vi "CRYImp wiz load settings.vi"() -> (0 "error out":errorcluster, 1 "Canceled":bool, 2 "x-y settings array out":T1 {"yp db ref" format="%.2f"; "ym db ref" format="%.2f"; "x db ref" format="%.2f"}, 3 "Main info cluster out":T2)   [LabVIEW 2013]
uses:
  Control/CRYImp wiz main info.ctl
  Control/CRYx-y settings array.ctl
  CRYMainGlobal.vi
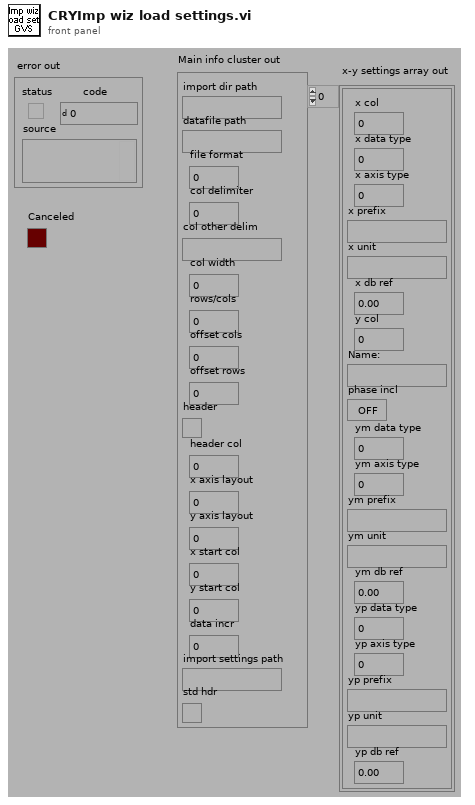
[diagram p1: front panel]
types:
  T1 = typedef "CRYx-y settings array.ctl" = cluster{"x col":i32, "x data type":u16, "x axis type":u16, "x prefix":string, "x unit":string, "x db ref":dbl, "y col":i32, "Name:":string, "phase incl":bool, "ym data type":u16, "ym axis type":u16, "ym prefix":string, "ym unit":string, "ym db ref":dbl, "yp data type":u16, "yp axis type":u16, "yp prefix":string, "yp unit":string, "yp db ref":dbl}[]
  T2 = typedef "CRYImp wiz main info.ctl" = cluster{"import dir path":path, "datafile path":path, "file format":i32, "col delimiter":i32, "col other delim":string, "col width":i32, "rows/cols":i32, "offset cols":i32, "offset rows":i32, "header":bool, "header col":i32, "x axis layout":i32, "y axis layout":i32, "x start col":i32, "y start col":i32, "data incr":i32, "import settings path":path, "std hdr":bool}
  T3 = enum32{"existing file", "new file", "new or existing file", "existing dir", "new dir", "new or existing dir", "existing file (use LLBs)", "new file (use LLBs)", "new or existing file (use LLBs)", "new or existing file or directory (use LLBs)", "existing dir (use LLBs)", "new dir (use LLBs)", "new or existing dir (use LLBs)", "existing file or dir", "new file or dir", "new or existing file or dir", "existing file or dir (use LLBs)", "new file or dir (use LLBs)"}
  T4 = enum16{"read/write", "read-only", "write-only", "write-only (truncate)"}
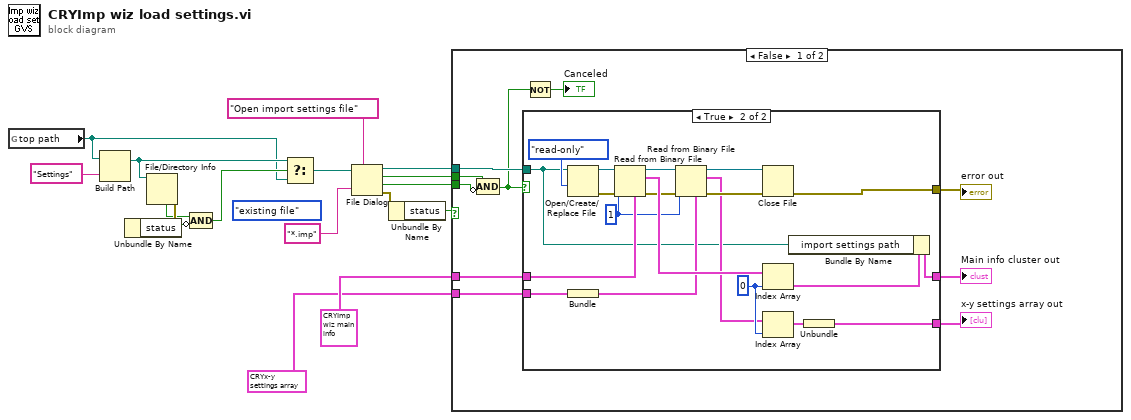
[diagram p0: block diagram]
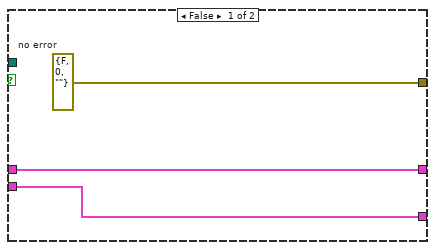
[diagram p2: hidden frame]
diagram:
  (unwired) T3."existing file" ("select mode (2)")
  n1 = global read "CRYMainGlobal.vi" "top path"() -> (w3:path)
  n2 = Build Path(base path=w3, name or relative path="Settings") -> (appended path=w5:path)
  n3 = File/Directory Info(path=w5) -> (directory=w7:bool, error out=w9:errorcluster)  [unwired: 1 in, 5 out]
  n4 = Unbundle By Name(w9) -> ("status"=w8:bool)
  n5 = Compound Arithmetic op=AND(w7, invert w8) -> (w6:bool)
  n6 = Select(t=w5, s=w6, f=w3) -> (s? t:f=w4:path)
  n7 = File Dialog(6:"*.imp" ("pattern"), 7:"Open import settings file" ("prompt"), 11:w4) -> (0:w2:errorcluster, 1:w14:bool, 2:w13:bool, 3:w12:path)  [unwired: 1 in, 3 out]
  n8 = Unbundle By Name(w2) -> ("status"=w1:bool)
  n9 = case shown="False" w1 {
    tunnel: w14 -> [w27 _]
    tunnel: w13 -> [w26 _]
    tunnel: w12 -> [w25 _]
    tunnel: T2 {"import dir path"=path "", "datafile path"=path "", "file format"=0, "col delimiter"=0, "col other delim"="", "col width"=0, "rows/cols"=0, "offset cols"=0, "offset rows"=0, "header"=FALSE, "header col"=0, "x axis layout"=0, "y axis layout"=0, "x start col"=0, "y start col"=0, "data incr"=0, "import settings path"=path "", "std hdr"=FALSE} ("Main info cluster out") -> [w24 _]
    tunnel: T1 [{"x col"=0, "x data type"=0, "x axis type"=0, "x prefix"="", "x unit"="", "x db ref"=0.0, "y col"=0, "Name:"="", "phase incl"=FALSE, "ym data type"=0, "ym axis type"=0, "ym prefix"="", "ym unit"="", "ym db ref"=0.0, "yp data type"=0, "yp axis type"=0, "yp prefix"="", "yp unit"="", "yp db ref"=0.0}] ("x-y settings array") -> [w19 _]
    frame False {
      n10 = Compound Arithmetic op=AND(w26, invert w27) -> (w21:bool)
      n11 = case shown="True" w21 {
        tunnel: w25 -> [_ w31]
        tunnel: w24 -> [w30 w49]
        tunnel: [w30 w32] -> w23
        tunnel: [w29 w45] -> w22
        tunnel: w19 -> [w28 w38]
        tunnel: [w28 w34] -> w18
        frame False {
          w29 = errorcluster {"status"=FALSE, "code"=0, "source"=""}  # no error
        }
        frame True {
          w39 = 0 ("Index")
          w40 = 1 ("count")
          n12 = Open/Create/Replace File(file path (use dialog)=w31, access (0:read/write)=T4."read-only" ("open mode (0)")) -> (refnum out=w47:refnum<file>, error out=w48:errorcluster)  [unwired: 1 in, 4 out]
          n13 = Bundle("x-y settings array"=w38) -> (w37:cluster{"x-y settings array":T1})  [unwired: 1 in]
          n14 = Read from Binary File(5:w49, 8:w48, 10:w40, 11:w47) -> (0:w43:errorcluster, 2:w46:T2[], 3:w44:refnum<file>)  [unwired: 3 out]
          n15 = Read from Binary File(5:w37, 8:w43, 10:w40, 11:w44) -> (0:w42:errorcluster, 2:w36:cluster{"x-y settings array":T1}[], 3:w41:refnum<file>)  [unwired: 3 out]
          n16 = Close File(refnum=w41, error in=w42) -> (error out=w45:errorcluster)  [unwired: 1 out]
          n17 = Index Array(array=w46, index=w39) -> (element=w33:T2)
          n18 = Index Array(array=w36, index=w39) -> (element=w35:cluster{"x-y settings array":T1})
          n19 = Bundle By Name(cluster=w33, "import settings path"=w31) -> (w32:T2)
          n20 = Unbundle(w35) -> ("x-y settings array"=w34:T1)
        }
      }
      "Main info cluster out" <- w23
      "error out" <- w22
      "x-y settings array out" <- w18
      n21 = Not(x=w21) -> (.not. x?=→"Canceled":bool)
    }
    frame True {
    }
  }
